vi "SDG60CreateArbWaveformFlatten.vi"(5 "WFM (Column) Number":i32, 6 "Array WFM":i16[](array[numeric])=[1000, 2000, 3000, 4000, 5000, 6000, 7000, 8000], 7 "WFM Length":i32=15, 8 "error in (no error)":errorcluster, 9 "Timeout (40000 ms)":u32=40000, 10 "Waveform Name (\"wave1\")":string="wave1", 11 "VISA resource name":refnum<visa-resource-name>="USB0::0xF4EC::0x1101::SDG6XEBC5R0119::INSTR") -> (0 "error out":errorcluster, 3 "VISA resource name out":refnum<visa-resource-name>)   [LabVIEW 2018]
doc: "Creates and saves an arbitrary (user-defined) waveform in non-volatile memory, then selects it for output."
uses:
  <vilib>/Utility/file.llb/Read From Spreadsheet File (I64).vi
panel:
  out "Flatten 2":string
  out "Orig Arr":string[](array[string])
  out "Concat":string
  out "Flatten":string
  out "Non-Matching Strings":bool
  out "WFM to arr time":dbl
  out "Arr to str time":dbl
  out "Upload time":dbl
  out "Total time":dbl
  out "Attempts":i32
  in  "WFM Source":u16(ring) items=["Single file", "Split files", "Array"]
  in  "WFM Path":path=path "C:/Data/_SoftDevelopment/SDG6000/data67107840.txt"
  # "Need to set name to be number. not string"
  # "Same vi as with suppliers example,\nbut incorrect negativ case removed.\nInstead calculating twos complement\nexplicitly for negative values.\nThe input range for ARB data is\n-32767..+32767"
  # "C1 hardcoded as needs to have a channel\nassigned to be uploaded. \nCan then be selected for either channel"
  # "Max  20E6 (decimal)"
  # "Need to reset device (*RST) to upload long (?) wavelength from PC to device\nFor now can't see another way to clear memory."
  # "Upon overwrite of name with new WFM, still needs to be selected\notherwise will still use old WFM. If WFM has been selected, and then gets deleted off \nC drive, will still output WFM on that channel"
  # "Testing uploads of large WFMS.\n8M: All ok, can have 2 separate WFMs on 2 channels and upload more\n16M: Can have 2 separate WFMs on 2 channels, storage space limits 3rd upload\n          of 16M points, but can upload 8M and switch fine between them all. Can't\n          upload an overwriting 16M point WFM when 2 already saved.\n20M: Can have 20M on both channels, but then no storage space to upload, need to delete\n          old waveform. Upon deletion, can upload 20M and select fine. \n          Could not do this yesterday, so may require more investigation.\n??? Is it possible to *RST and then overwrite without deleting wfms manually?\nIf too large a waveform is uploaded, generator will crash requiring manual power cycle"
  # "If storage full, will beep on \nmachine-say storage full, \nbut not give any error through \nlabview. Waveform won't ovewrite\nothers when uploading"
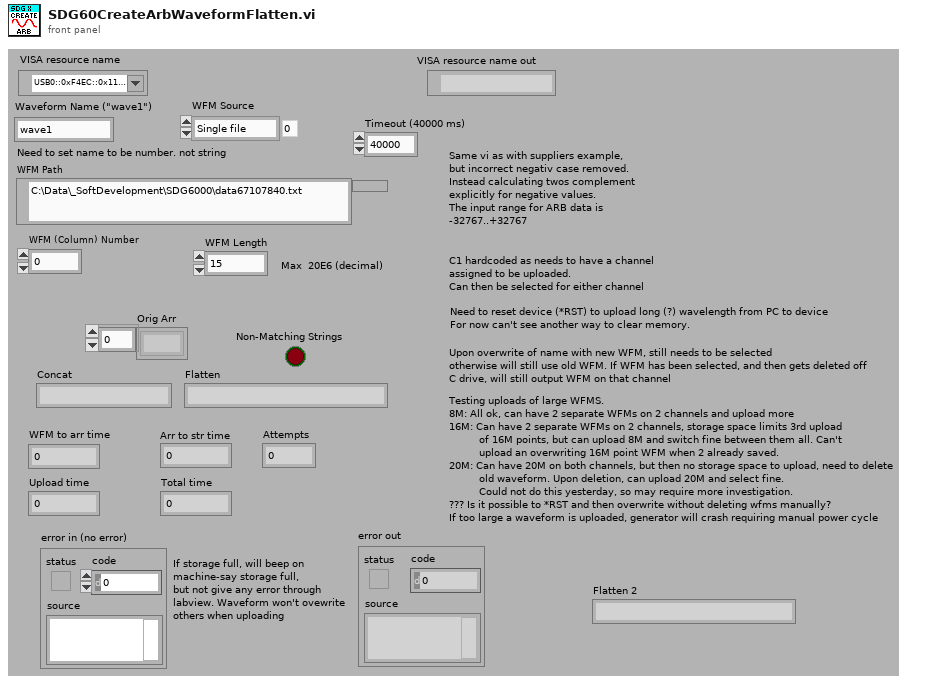
[diagram p1: front panel]
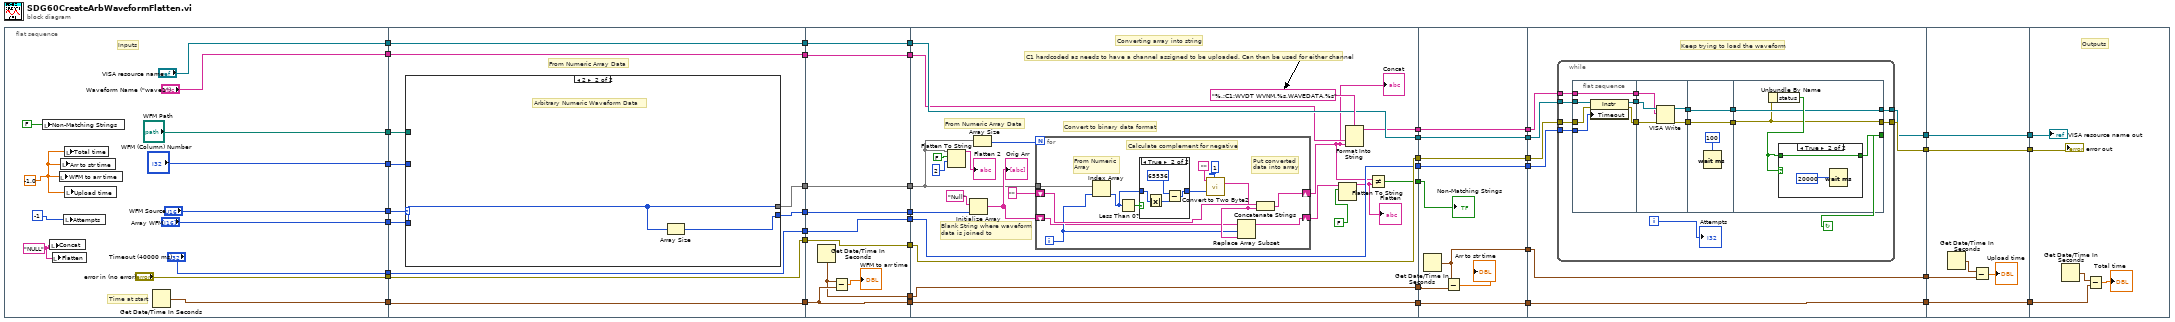
[diagram p0: block diagram]
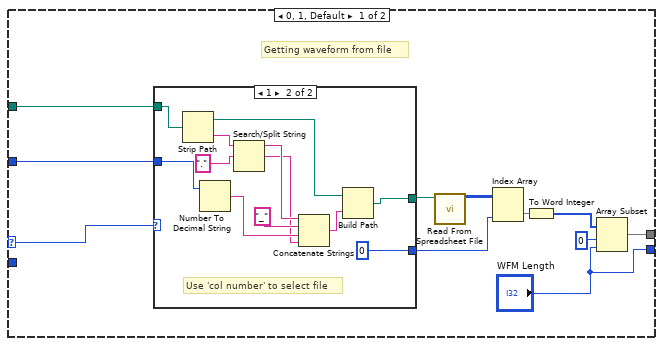
[diagram p2: hidden frame]
diagram:
  n1 = flat-sequence {
    tunnel: ["WFM Source"] -> w44
    tunnel: ["Array WFM"] -> w43
    tunnel: ["WFM Path"] -> w42
    tunnel: ["WFM (Column) Number"] -> w41
    tunnel: ["VISA resource name"] -> w40
    tunnel: ["Waveform Name (\"wave1\")"] -> w39
    tunnel: ["error in (no error)"] -> w38
    tunnel: ["Timeout (40000 ms)"] -> w37
    tunnel: [w49] -> w36
    tunnel: w44 -> [w68]
    tunnel: w43 -> [w67]
    tunnel: [w66] -> w35
    tunnel: w42 -> [w65]
    tunnel: w41 -> [w64]
    tunnel: [w63] -> w33
    tunnel: w40 -> [w63]
    tunnel: [w62] -> w31
    tunnel: w39 -> [w62]
    tunnel: [w61] -> w29
    tunnel: w38 -> [w61]
    tunnel: [w60] -> w27
    tunnel: w37 -> [w60]
    tunnel: [w59] -> w25
    tunnel: w36 -> [w59]
    tunnel: [w58] -> w1
    tunnel: w35 -> [w104]
    tunnel: [w104] -> w34
    tunnel: w33 -> [w103]
    tunnel: [w103] -> w32
    tunnel: w31 -> [w102]
    tunnel: [w102] -> w30
    tunnel: w29 -> [w98]
    tunnel: [w98] -> w28
    tunnel: w27 -> [w99]
    tunnel: [w99] -> w26
    tunnel: w25 -> [w100]
    tunnel: [w100] -> w24
    tunnel: [w97] -> w4
    tunnel: [w96] -> w2
    tunnel: w1 -> [w96]
    tunnel: w34 -> [w107]
    tunnel: [w115] -> w23
    tunnel: [w123] -> w21
    tunnel: [w122] -> w19
    tunnel: [w121] -> w17
    tunnel: w32 -> [w123]
    tunnel: w30 -> [w120]
    tunnel: w28 -> [w122]
    tunnel: w26 -> [w121]
    tunnel: w24 -> [w119]
    tunnel: [w119] -> w15
    tunnel: [w118] -> w5
    tunnel: w4 -> [w118]
    tunnel: [w116] -> w3
    tunnel: w2 -> [w109]
    tunnel: w23 -> [w152]
    tunnel: [w152] -> w22
    tunnel: w21 -> [w151]
    tunnel: [w151] -> w20
    tunnel: w19 -> [w150]
    tunnel: [w150] -> w18
    tunnel: w17 -> [w149]
    tunnel: [w149] -> w16
    tunnel: w15 -> [w145]
    tunnel: [w145] -> w14
    tunnel: [w147] -> w7
    tunnel: w5 -> [w146]
    tunnel: w3 -> [w144]
    tunnel: [w156] -> w13
    tunnel: [w155] -> w11
    tunnel: w22 -> [w160]
    tunnel: w20 -> [w159]
    tunnel: w18 -> [w158]
    tunnel: w16 -> [w157]
    tunnel: w14 -> [w154]
    tunnel: [w154] -> w9
    tunnel: w7 -> [w153]
    tunnel: [w153] -> w6
    tunnel: w13 -> [w202]
    tunnel: [w202] -> w12
    tunnel: w11 -> [w201]
    tunnel: [w201] -> w10
    tunnel: w9 -> [w199]
    tunnel: [w199] -> w8
    tunnel: w6 -> [w198]
    tunnel: w12 -> [w207]
    tunnel: w10 -> [w206]
    tunnel: w8 -> [w203]
    frame #0 {
      w45 = "NULL"
      w48 = -1.0
      # "Inputs"
      # "Time at start"
      n2 = local write "Non-Matching Strings"(FALSE) -> ()
      n3 = local write "Concat"(w45) -> ()
      n4 = local write "Flatten"(w45) -> ()
      n5 = local write "WFM to arr time"(w48) -> ()
      n6 = local write "Arr to str time"(w48) -> ()
      n7 = local write "Attempts"(-1) -> ()
      n8 = local write "Total time"(w48) -> ()
      n9 = local write "Upload time"(w48) -> ()
      n10 = Get Date/Time In Seconds() -> (seconds since 1Jan1904=w49:timestamp)
    }
    frame #1 {
      # "From Numeric Array Data"
      n11 = case shown="2" w68 {
        selector: w68 -> [w77 _]
        tunnel: [w72 w95] -> w66
        tunnel: w67 -> [_ w95]
        tunnel: w65 -> [w71 _]
        tunnel: w64 -> [w70 _]
        tunnel: ["WFM Length" w94] -> w58
        frame 0, 1, Default {
          # "Getting waveform from file"
          n12 = case shown="1" w77 {
            tunnel: w71 -> [w81 w93]
            tunnel: w70 -> [w80 w90]
            tunnel: [w81 w83] -> w75
            tunnel: [w80 0 ("x")] -> w74
            frame 0, Default {
              # "File contains multiple wfms"
            }
            frame 1 {
              # "Use 'col number' to select file"
              n13 = Strip Path(path=w93) -> (stripped path=w85:path, name=w91:string)
              n14 = Number To Decimal String(number=w90) -> (decimal integer string=w87:string)  [unwired: 1 in]
              n15 = Search/Split String(string=w91, search string/char (-)=".") -> (substring before match=w89:string, match + rest of string=w86:string)  [unwired: 1 in, 1 out]
              n16 = Concatenate Strings(w89, "_", w87, w86) -> (w84:string)
              n17 = Build Path(base path=w85, name or relative path=w84) -> (appended path=w83:path)
            }
          }
          n18 = call-poly <vilib>:"Read From Spreadsheet File.vi"("file path (dialog if empty)"=w75) -> ("all rows"=w76:i64[][])  [unwired: 6 in, 4 out]
          n19 = Index Array(array=w76, index (col)=w74) -> (element=w73:i64[])  [unwired: 1 in]
          n20 = To Word Integer(number=w73) -> (16bit integer=w79:i16[])
          n21 = Array Subset(array=w79, index=0 ("x"), length="WFM Length") -> (w72:i16[])
        }
        frame 2 {
          # "Arbitrary Numeric Waveform Data"
          n22 = Array Size(array=w95) -> (size(s)=w94:i32)
        }
      }
    }
    frame #2 {
      n23 = Get Date/Time In Seconds() -> (seconds since 1Jan1904=w97:timestamp)
      n24 = Subtract(x=w97, y=w100) -> (x-y=→"WFM to arr time":dbl)
    }
    frame #3 {
      # "Converting array into string"
      # "Blank String where waveform\ndata is joined to"
      # "C1 hardcoded as needs to have a channel assigned to be uploaded. Can then be used for either channel"
      # "From Numeric Array Data"
      # "Convert to binary data format"
      n25 = Flatten To String(anything=w107, prepend array or string size? (T)=FALSE, byte order (0:big-endian, network order)=2) -> (data string=→"Flatten 2":string)  [unwired: 1 in, 2 out]
      n26 = Initialize Array("Null", w109) -> (w111:string[])
      "Orig Arr" <- w111
      n27 = Array Size(array=w107) -> (size(s)=w125:i32)
      n28 = for {
        N: w125 -> [_]
        shift-right: [w133] -> w114
        shift-left: "" -> [w132]
        tunnel: w107 -> [w131]
        shift-right: [w127] -> w112
        shift-left: w111 -> [w128]
        i -> [w129]
        # "Calculate complement for negative"
        # "From Numeric\nArray"
        # "Put converted\ndata into array"
        n29 = Index Array(array=w131, index=w129) -> (element=w135:i16)
        n30 = Less Than 0?(x=w135) -> (x < 0?=w136:bool)
        n31 = case shown="True" w136 {
          tunnel: w135 -> [w139 w140]
          tunnel: [w139 w143] -> w134
          frame False {
          }
          frame True {
            n32 = Absolute Value(x=w140) -> (abs(x)=w141:i16)
            n33 = Subtract(x=65536, y=w141) -> (x-y=w143:i32)
          }
        }
        n34 = call "Convert to Two Byte2.vi"("Input Method (0:String)"=u16 1, "Input Number"=w134, "Numeric String"="") -> ("Output String"=w130:string)  [unwired: 8 in]
        n35 = Replace Array Subset(array=w128, new element=w130, index=w129) -> (w127:string[])
        n36 = Concatenate Strings(w132, w130) -> (w133:string)
      }
      "Concat" <- w114
      n37 = Flatten To String(anything=w112, prepend array or string size? (T)=FALSE) -> (data string=w110:string)  [unwired: 2 in, 2 out]
      "Flatten" <- w110
      n38 = Format Into String(format string="%.;C1:WVDT WVNM,%s,WAVEDATA,%s", w120, w114) -> (resulting string=w115:string)  [unwired: 2 in, 1 out]
      n39 = Not Equal?(x=w114, y=w110) -> (x != y?=w116:bool)
    }
    frame #4 {
      n40 = Get Date/Time In Seconds() -> (seconds since 1Jan1904=w147:timestamp)
      n41 = Subtract(x=w147, y=w146) -> (x-y=→"Arr to str time":dbl)
      "Non-Matching Strings" <- w144
    }
    frame #5 {
      # "Keep trying to load the waveform"
      n42 = while {
        tunnel: w160 -> [w175]
        tunnel: w159 -> [w174]
        tunnel: w158 -> [w173]
        tunnel: [w172] -> w156
        tunnel: [w171] -> w155
        tunnel: w157 -> [w161]
        i -> [w167]
        stop <- w170 continue-if-true
        n43 = flat-sequence {
          tunnel: w175 -> [w181]
          tunnel: w173 -> [w178]
          tunnel: w174 -> [w180]
          tunnel: [w179] -> w164
          tunnel: [w177] -> w163
          tunnel: [w181] -> w162
          tunnel: w161 -> [w176]
          tunnel: [w182] -> w169
          tunnel: [w183] -> w168
          tunnel: w164 -> [w185]
          tunnel: w163 -> [w186]
          tunnel: w162 -> [w184]
          tunnel: w169 -> [w187]
          tunnel: w168 -> [w188]
          tunnel: [w188] -> w166
          tunnel: [w187] -> w165
          tunnel: [w191] -> w171
          tunnel: [w190] -> w172
          tunnel: [w192] -> w170
          tunnel: w166 -> [w191]
          tunnel: w165 -> [w190]
          frame #0 {
            n44 = property class="Instr"(reference=w180, error in=w178, "Timeout"=w176) -> (reference out=w179:refnum<visa-resource-name>, error out=w177:errorcluster)
          }
          frame #1 {
            n45 = VISA Write(VISA resource name=w185, write buffer=w184, error in (no error)=w186) -> (VISA resource name out=w183:refnum<visa-resource-name>, error out=w182:errorcluster)  [unwired: 1 out]
          }
          frame #2 {
            n46 = Wait (ms)(milliseconds to wait=100 ("x")) -> ()  [unwired: 1 out]
          }
          frame #3 {
            n47 = Unbundle By Name(w190) -> ("status"=w193:bool)
            n48 = case shown="True" w193 {
              tunnel: w193 -> [w194 w195]
              tunnel: [w194 w195] -> w192
              frame False {
              }
              frame True {
                n49 = Wait (ms)(milliseconds to wait=20000 ("x")) -> ()  [unwired: 1 out]
              }
            }
          }
        }
        "Attempts" <- w167
      }
    }
    frame #6 {
      n50 = Get Date/Time In Seconds() -> (seconds since 1Jan1904=w200:timestamp)
      n51 = Subtract(x=w200, y=w198) -> (x-y=→"Upload time":dbl)
    }
    frame #7 {
      # "Outputs"
      n52 = Get Date/Time In Seconds() -> (seconds since 1Jan1904=w205:timestamp)
      n53 = Subtract(x=w205, y=w203) -> (x-y=→"Total time":dbl)
      "VISA resource name out" <- w206
      "error out" <- w207
    }
  }
